vi "List All Methods.vi"() -> (3 "All Methods":string)   [LabVIEW 2019, in "HTTP Server.lvlib"]
uses:
  HTTP Server.lvlib
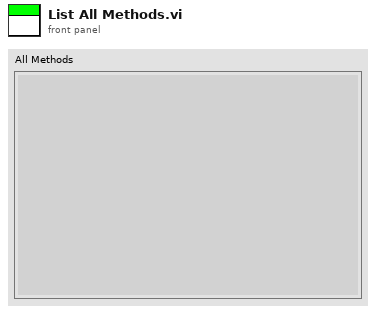
[diagram p1: front panel]
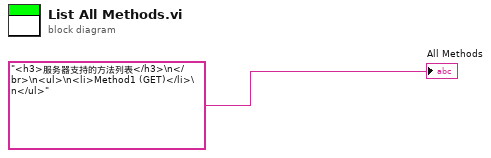
[diagram p0: block diagram]
diagram:
  "All Methods" <- "<h3>服务器支持的方法列表</h3>\n</br>\n<ul>\n<li>Method1 (GET)</li>\n</ul>" ("All Methods")
